vi "TrackPupil.vi"(4 "Processed image display refnum":T1, 5 "Processed image":T1, 6 "Mask refnum":T1, 7 "Fitted image refnum":T1, 8 "Circle fit parameters in":T3, 9 "Rescan image if pupil is lost":bool=TRUE, 10 "Acquired image refnum":T1, 11 "Cropped image refnum":T1) -> (0 "Circle fit parameters out":T3, 1 "New Values":T2, 2 "Processed image display refnum out":T1, 3 "Fitted image refnum out":T1)   [LabVIEW 2013]
doc: "Fit a circle to identified pupil in the cropped image and update Circle fit parameters. Also overlays a circle on the original image.\n\nInputs/outputs\n\nAcquired image refnum - Original image acquired from camera\n\nProcessed image refnum - Cropped image which is thresholded and processed before circular fitting to pupil\n\nCropped image refnum - Cropped version of original image\n\nManual Threshold (array) - lower and upper limits for thresholding of the cropped image\n\nCircle fit parameters (cluster of 5 elements)\n - Frame No (int) - Number of the current frame\n - Circle Time series (array) - A table for storing results from circle fitting, e.g frame no, radius and x and y coordinates for center position\n - Rectangle coordinates (array) - Rectangle coordinates for the cropped region of the picture\n - Annulus ROI (cluster) - An annulus ROI from the imaq package\n - Annulus coordinates (array) - Annulus coordinates of the Annulus ROI"
uses:
  <vilib>/vision/Image Controls.llb/IMAQ Image.ctl
  TrackingParameters.ctl
  <vilib>/vision/NI_Vision_Development_Module.lvlib
panel:
  # "Fit a circle to identified pupil in the cropped image and update Circle fit parameters. Also overlays a circle on the original image."
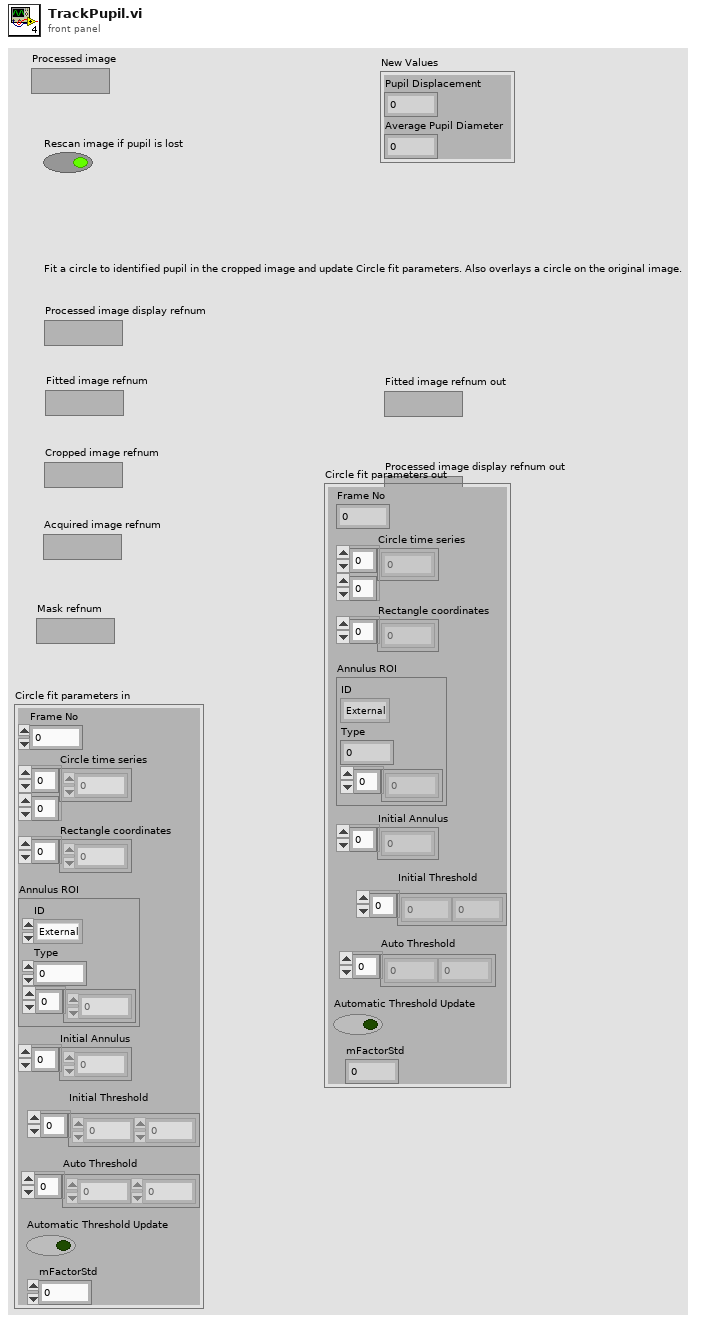
[diagram p1: front panel]
types:
  T1 = typedef "IMAQ Image.ctl" = refnum<image>
  T2 = cluster{"Pupil Displacement":dbl, "Average Pupil Diameter":dbl}
  T3 = typedef "TrackingParameters.ctl" = cluster{"Frame No":i32, "Circle time series":dbl[][], "Rectangle coordinates":i32[], "Annulus ROI":cluster{"ID":enum32{"External", "Internal"}, "Type":u32, i32[]}, "Initial Annulus":i32[], "Auto Threshold":sgl[], "Automatic Threshold Update":bool, "Initial Threshold":sgl[], "mFactorStd":dbl}
  T4 = cluster{"Global Rectangle":i32[], "Contours":cluster{"ID":enum32{"External", "Internal"}, "Type":u32, "Coordinates":i32[]}[]}
  T5 = cluster{"Process":enum16{"Get First Edge", "Get First + Last Edge", "Get All Edges", "Get Best Edge"}, "Step Size":i32, "Max Pixel Radius":i32}
  T6 = cluster{"ID":enum32{"External", "Internal"}, "Type":u32, i32[]}
  T7 = cluster{"ID":enum32{"External", "Internal"}, "Type":u32, i32[]}[]
  T8 = cluster{"Center (Pixels)":cluster{"X":sgl, "Y":sgl}, "Radius (Pixels)":dbl, "Center (Real-World)":cluster{"X":sgl, "Y":sgl}, "Radius (Real-World)":dbl, "Roundness (Real-World)":dbl, "Average Strength":dbl, "Average SNR (dB)":dbl}
  T9 = typedef "IMAQ Circle" = cluster{"Center X":i32, "Center Y":i32, "Inner Radius":i32, "Outer Radius":i32, "Start Angle":dbl, "End Angle":dbl}
  T10 = typedef "ROI Descriptor" = cluster{"Global Rectangle":i32[], "Contours":cluster{"ID":enum32{"External", "Internal"}, "Type":u32, "Coordinates":i32[]}[]}
  T11 = cluster{"histogram":u32[], "Minimal Value":sgl, "Maximal Value":sgl, "Starting Value":sgl, "Interval Width":sgl, "Mean Value":sgl, "Standard  Variation":sgl, "Area (pixels)":i32}
  T12 = cluster{"Rectangle[0]":i32, "Rectangle[1]":i32, "Rectangle[2]":i32, "Rectangle[3]":i32}
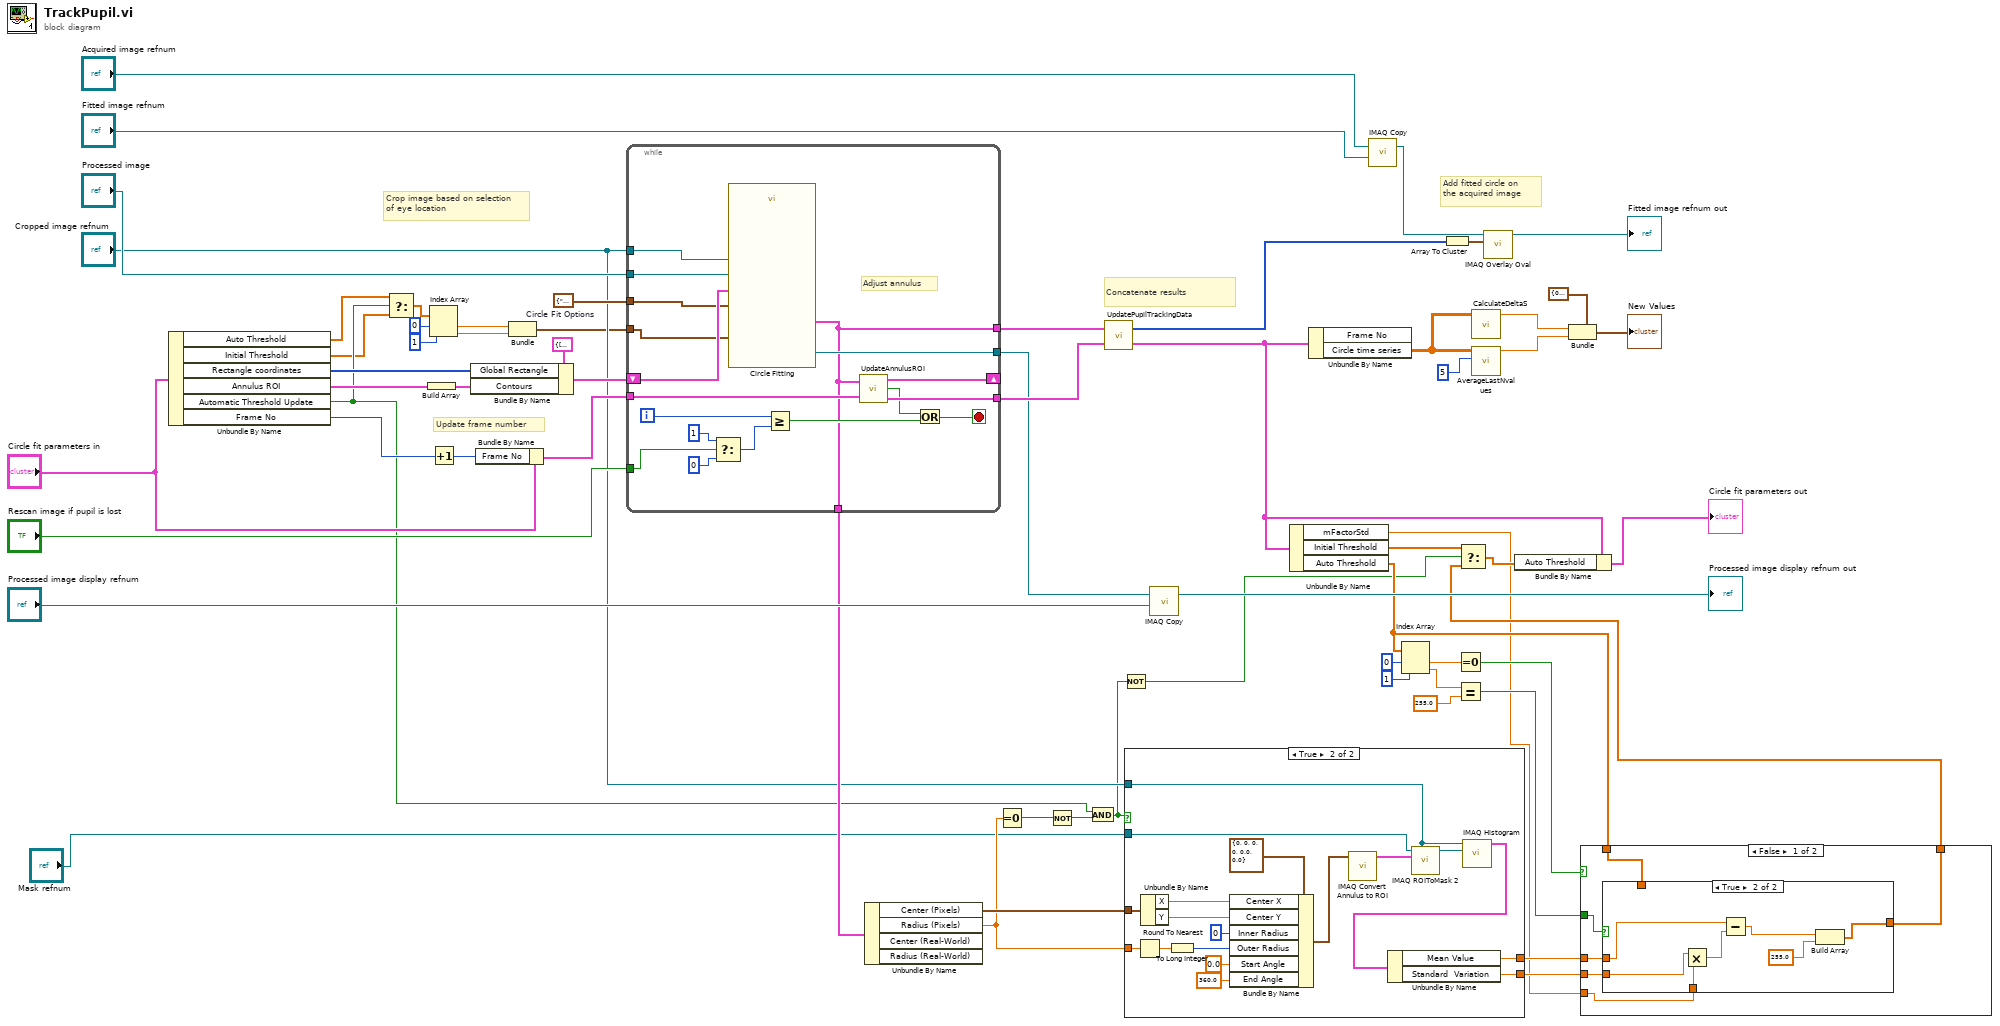
[diagram p0: block diagram]
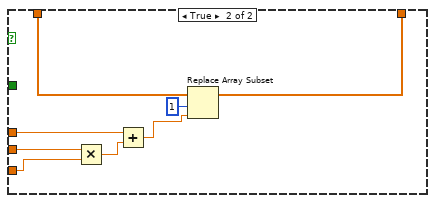
[diagram p3: hidden frame]
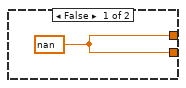
[diagram p4: hidden frame]
diagram:
  w58 = T5 {"Process"=enum."Get First Edge", "Step Size"=16, "Max Pixel Radius"=5}  # Circle Fit Options
  # "Update frame number"
  # "Add fitted circle on the acquired image"
  # "Crop image based on selection of eye location"
  # "Concatenate results"
  n1 = Unbundle By Name("Circle fit parameters in") -> ("Auto Threshold"=w14:sgl[], "Initial Threshold"=w13:sgl[], "Rectangle coordinates"=w51:i32[], "Annulus ROI"=w50:T6, "Automatic Threshold Update"=w15:bool, "Frame No"=w17:i32)
  n2 = Select(t=w14, s=w15, f=w13) -> (s? t:f=w12:sgl[])
  n3 = Build Array(w50) -> (w57:T7)
  n4 = Index Array(array=w12, index #1=0 ("index"), index #2=1 ("index")) -> (element #1=w9:sgl, element #2=w8:sgl)
  n5 = Increment(x=w17) -> (x+1=w16:i32)
  n6 = Bundle By Name(cluster=T4 {"Global Rectangle"=[63, 39, 363, 338], "Contours"=[{"ID"=enum."External", "Type"=7, "Coordinates"=[212, 188, 9, 149, 0, 0]}]} ("ROI Descriptor (Find Circular Edge 1)"), "Global Rectangle"=w51, "Contours"=w57) -> (w60:T4)
  n7 = Bundle By Name(cluster="Circle fit parameters in", "Frame No"=w16) -> (w55:T3)
  n8 = Bundle("Numeric"=w9, "Numeric"=w8) -> (w7:cluster{"Numeric":sgl, "Numeric":sgl})  [unwired: 1 in]
  n9 = while {
    tunnel: [w81] -> w37
    tunnel: w7 -> [w64]
    tunnel: "Cropped image refnum" -> [w80]
    tunnel: w58 -> [w78]
    tunnel: [w65] -> w53
    tunnel: w55 -> [w75]
    tunnel: [w74] -> w54
    shift-right: [w71] -> _
    shift-left: w60 -> [w79]
    tunnel: "Rescan image if pupil is lost" -> [w67]
    tunnel: "Processed image" -> [w66]
    tunnel: [w65] -> w36
    i -> [w77]
    stop <- w76 stop-if-true
    # "Adjust annulus"
    n10 = Select(t=1, s=w67, f=0) -> (s? t:f=w70:i32)
    n11 = call "Circle Fitting"("Image In"=w80, "Range (Threshold 2)"=w64, "ROI Descriptor (Find Circular Edge 1)"=w79, "Circle Fit Options (Find Circular Edge 1)"=w78, "Image Dst"=w66) -> ("Image Out"=w81:T1, "Fitted Circle (Find Circular Edge 1)"=w65:T8)  [unwired: 20 in, 1 out]
    n12 = Greater Or Equal?(x=w77, y=w70) -> (x >= y?=w73:bool)
    n13 = call "UpdateAnnulusROI.vi"("Fitted Circle"=w65, "Circle fit parameters in"=w75) -> ("Annulus Roi"=w71:T4, "Pupil Found"=w72:bool, "Circle fit parameters out"=w74:T3)
    n14 = Or(x=w72, y=w73) -> (x .or. y?=w76:bool)
  }
  n15 = Unbundle By Name(w36) -> ("Center (Pixels)"=w35:cluster{"X":sgl, "Y":sgl}, "Radius (Pixels)"=w33:dbl)  [unwired: 2 out]
  n16 = Equal To 0?(x=w33) -> (x = 0?=w5:bool)
  n17 = Not(x=w5) -> (.not. x?=w4:bool)
  n18 = And(x=w15, y=w4) -> (x .and. y?=w3:bool)
  n19 = call "UpdatePupilTrackingData.vi"("Circle fit parameters in"=w54, "Fitted Circle"=w53) -> ("Circle fit parameters out"=w31:T3, "Rectangle"=w61:i32[])
  n20 = Not(x=w3) -> (.not. x?=w2:bool)
  n21 = case shown="True" w3 {
    tunnel: w35 -> [_ w95]
    tunnel: "Cropped image refnum" -> [_ w92]
    tunnel: w33 -> [_ w90]
    tunnel: [w82 w89] -> w24
    tunnel: [w82 w88] -> w23
    tunnel: "Mask refnum" -> [_ w83]
    frame False {
      w82 = sgl nan ("Mean Value")
    }
    frame True {
      n22 = Round To Nearest(number=w90) -> (nearest integer value=w96:dbl)
      n23 = Unbundle By Name(w95) -> ("X"=w94:sgl, "Y"=w93:sgl)
      n24 = To Long Integer(number=w96) -> (32bit integer=w97:i32)
      n25 = Bundle By Name(cluster=T9 {"Center X"=0, "Center Y"=0, "Inner Radius"=0, "Outer Radius"=0, "Start Angle"=0.0, "End Angle"=0.0} ("Annulus"), "Center X"=w94, "Center Y"=w93, "Inner Radius"=0, "Outer Radius"=w97, "Start Angle"=0.0, "End Angle"=360.0) -> (w86:T9)
      n26 = call "IMAQ Convert Annulus to ROI"("Annulus"=w86) -> ("ROI Descriptor"=w100:T10)  [unwired: 8 in, 1 out]
      n27 = call "IMAQ ROIToMask 2"("Image Model"=w92, "ROI Descriptor"=w100, "Image"=w83) -> ("Image Out"=w91:T1)  [unwired: 6 in, 2 out]
      n28 = call "IMAQ Histogram"("Image Mask"=w91, "Image"=w92) -> ("Histogram Report"=w87:T11)  [unwired: 8 in, 1 out]
      n29 = Unbundle By Name(w87) -> ("Mean Value"=w89:sgl, "Standard  Variation"=w88:sgl)
    }
  }
  n30 = call "IMAQ Copy"("Image Dst"="Processed image display refnum", "Image Src"=w37) -> ("Image Dst Out"=→"Processed image display refnum out":T1)  [unwired: 4 in, 1 out]
  n31 = Unbundle By Name(w31) -> ("mFactorStd"=w1:dbl, "Initial Threshold"=w20:sgl[], "Auto Threshold"=w21:sgl[])
  n32 = Unbundle By Name(w31) -> ("Circle time series"=w43:dbl[][])  [unwired: 1 out]
  n33 = call "IMAQ Copy"("Image Dst"="Fitted image refnum", "Image Src"="Acquired image refnum") -> ("Image Dst Out"=w45:T1)  [unwired: 4 in, 1 out]
  n34 = Index Array(array=w21, index #1=0 ("index"), index #2=1 ("index")) -> (element #1=w28:sgl, element #2=w27:sgl)
  n35 = Array To Cluster(array=w61) -> (cluster=w62:T12)
  n36 = Equal To 0?(x=w28) -> (x = 0?=w25:bool)
  n37 = Equal?(x=w27, y=sgl 255.0) -> (x = y?=w22:bool)
  n38 = call "CalculateDeltaS.vi"("Circle time series"=w43) -> ("Pupil Displacement"=w42:dbl)  [unwired: 10 in]
  n39 = call "AverageLastNvalues.vi"("N"=5, "Circle time series"=w43) -> ("Average of last N array elements"=w41:dbl)  [unwired: 9 in]
  n40 = call "IMAQ Overlay Oval"("Bounding Rectangle"=w62, "Image"=w45) -> ("Image Out"=→"Fitted image refnum out":T1)  [unwired: 8 in, 1 out]
  n41 = Bundle(cluster=T2 {"Pupil Displacement"=0.0, "Average Pupil Diameter"=0.0}, "Pupil Displacement"=w42, "Average Pupil Diameter"=w41) -> (→"New Values":T2)
  n42 = case shown="False" w25 {
    tunnel: w24 -> [w105 w122]
    tunnel: w23 -> [w104 w121]
    tunnel: w22 -> [w106 _]
    tunnel: w21 -> [w103 w119]
    tunnel: [w102 w117] -> w18
    tunnel: w1 -> [w101 w115]
    frame False {
      n43 = case shown="True" w106 {
        tunnel: w105 -> [_ w113]
        tunnel: w104 -> [_ w112]
        tunnel: w103 -> [w107 _]
        tunnel: [w107 w111] -> w102
        tunnel: w101 -> [_ w108]
        frame False {
        }
        frame True {
          n44 = Multiply(x=w112, y=w108) -> (x*y=w114:dbl)
          n45 = Subtract(x=w113, y=w114) -> (x-y=w110:dbl)
          n46 = Build Array(w110, sgl 255.0 ("element")) -> (w111:dbl[])
        }
      }
    }
    frame True {
      n47 = Multiply(x=w121, y=w115) -> (x*y=w120:dbl)
      n48 = Add(x=w122, y=w120) -> (x+y=w118:dbl)
      n49 = Replace Array Subset(array=w119, new element=w118, index=1) -> (w117:sgl[])
    }
  }
  n50 = Select(t=w20, s=w2, f=w18) -> (s? t:f=w19:dbl[])
  n51 = Bundle By Name(cluster=w31, "Auto Threshold"=w19) -> (→"Circle fit parameters out":T3)
